vi "FGV _Operator Name.vi"(10 "Enum":enum16{"Write", "Read"}(ring)=enum."Read", 11 "Operator Name in":string) -> (3 "Operator Name out":string)   [LabVIEW 2018, in "Application.lvlib"]
uses:
  Application.lvlib
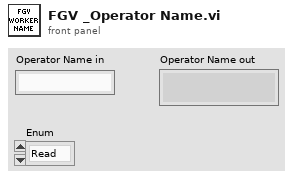
[diagram p1: front panel]
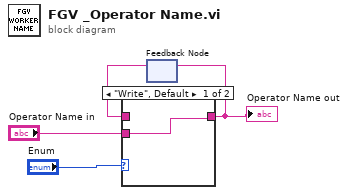
[diagram p0: block diagram]
diagram:
  n1 = feedback #1() -> (w3:string)  [unwired: 1 in]
  n2 = case shown="\"Write\", Default" "Enum" {
    tunnel: w3 -> [_ w6]
    tunnel: [w5 w6] -> w1
    tunnel: "Operator Name in" -> [w5 _]
    frame "Write", Default {
    }
    frame "Read" {
    }
  }
  "Operator Name out" <- w1
  n3 = feedback-in #1(w1) -> ()
